vi "set_cursor_pos.vi"(1 "y position":i32=200, 2 "x position":i32=200) -> ()   [LabVIEW 2014]
doc: "This Set Cursor Position VI sets the position of the mouse cursor on the screen programmatically. The VI uses the Call Library Function Node to call the Windows SDK function SetCursorPos. \n\nYou can modify the Set Cursor Position VI to position the mouse cursor programmatically in LabVIEW. In this example, select the horizontal pixel position of the cursor using the x position control. Use the y position control to select the vertical pixel position of the cursor."
uses:
  User32.dll
panel:
  # "Select Help»Show Context Help and move the cursor \nover the VI icon to display help for this VI."
  # "1) Set desired cursor   \n    position with \n    x position and \n    y position controls.\n2) Run VI"
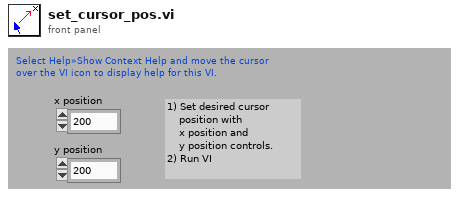
[diagram p1: front panel]
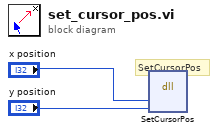
[diagram p0: block diagram]
diagram:
  # "SetCursorPos"
  n1 = dll-call lib="User32.dll" fn="SetCursorPos"("x position", "y position") -> ()  [unwired: 6 in, 2 out]
